vi "Remove Section.vi"(7 "Section Name":string, 8 "error in (no error)":errorcluster, 11 "Config in":refnum<class "LabVIEW-Config.lvclass">) -> (0 "error out":errorcluster, 2 "Section Found?":bool, 3 "Config out":refnum<class "LabVIEW-Config.lvclass">)   [LabVIEW 2017, in "LabVIEW-Config.lvlib" / "LabVIEW-Config.lvclass"]
uses:
  LabVIEW-Config.lvclass
  LabVIEW-Config.lvclass/LabVIEW-Config.ctl
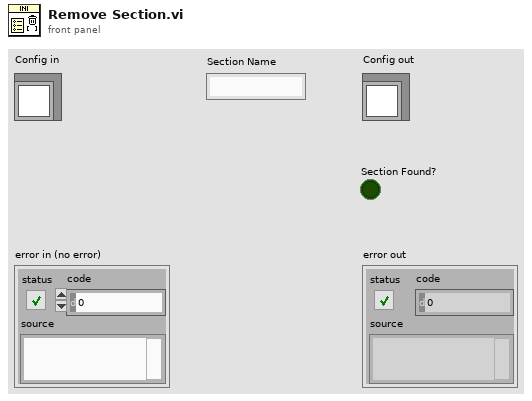
[diagram p1: front panel]
types:
  T1 = typedef "LabVIEW-Config.lvlib/LabVIEW-Config.lvclass/LineToken.ctl" = enum8{"comment", "section", "key", "more"}
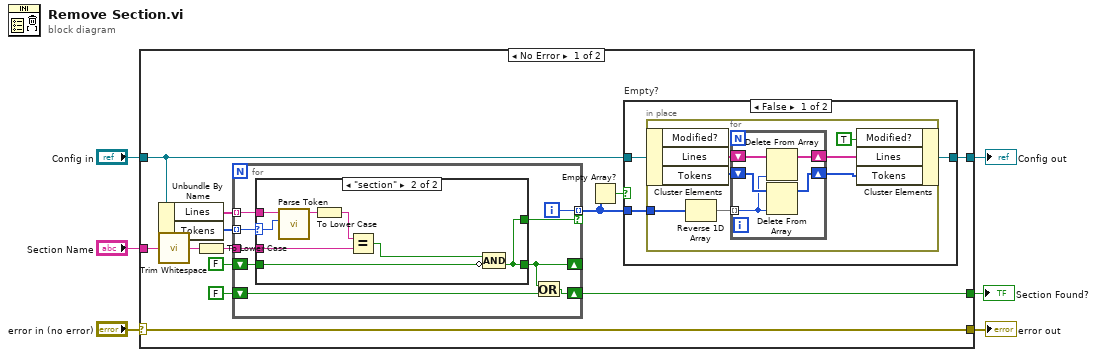
[diagram p0: block diagram]
diagram:
  n1 = case shown="No Error" "error in (no error)" {
    selector: "error in (no error)" -> [w17 w55]
    tunnel: "Config in" -> [w10 w54]
    tunnel: [w17 w55] -> w5
    tunnel: [w11 w54] -> w3
    tunnel: "Section Name" -> [w16 _]
    tunnel: [w12 _] -> w1
    frame No Error {
      n2 = Unbundle By Name(w10) -> ("Lines"=w18:string[], "Tokens"=w19:T1[])
      n3 = call <vilib>:"Trim Whitespace.vi"("string"=w16) -> ("trimmed string"=w7:string)  [unwired: 1 in]
      n4 = To Lower Case(string=w7) -> (all lower case string=w15:string)
      n5 = for {
        tunnel: w19 -> [w28] mode=indexing
        tunnel: w18 -> [w27] mode=indexing
        tunnel: [w20] -> w9 mode=indexing if=w24
        tunnel: w15 -> [w26]
        shift-right: [w23] -> _
        shift-left: FALSE -> [w25]
        shift-right: [w22] -> w12
        shift-left: FALSE -> [w21]
        i -> [w20]
        n6 = case shown="\"section\"" w28 {
          selector: w28 -> [_ w31]
          tunnel: w27 -> [_ w32]
          tunnel: w26 -> [_ w37]
          tunnel: [w29 w33] -> w23
          tunnel: w25 -> [w29 w35]
          tunnel: [w29 w33] -> w24
          frame Default {
          }
          frame "section" {
            n7 = call "Parse Token.vi"("Token"=w31, "Line"=w32) -> ("Name"=w30:string)  [unwired: 8 in, 1 out]
            n8 = To Lower Case(string=w30) -> (all lower case string=w36:string)
            n9 = Equal?(x=w36, y=w37) -> (x = y?=w34:bool)
            n10 = Compound Arithmetic op=AND(w34, invert w35) -> (w33:bool)
          }
        }
        n11 = Or(x=w23, y=w21) -> (x .or. y?=w22:bool)
      }
      n12 = Empty Array?(array=w9) -> (empty?=w8:bool)
      n13 = case "Empty?" shown="False" w8 {
        tunnel: [w40 w53] -> w11
        tunnel: w10 -> [w39 w53]
        tunnel: w9 -> [w38 _]
        frame False {
          n14 = in-place {
            in-place-border: w38 -> [w46]
            n15 = in-place-cluster #1(w39) -> ("Lines"=w45:string[], "Tokens"=w44:T1[])  [unwired: 1 out]
            n16 = Reverse 1D Array(array=w46) -> (reversed array=w41:i32[])
            n17 = for {
              shift-right: [w51] -> w42
              shift-left: w45 -> [w52]
              shift-right: [w48] -> w43
              shift-left: w44 -> [w50]
              tunnel: w41 -> [w49] mode=indexing
              n18 = Delete From Array(array=w52, index=w49) -> (array with subset deleted=w51:string[])  [unwired: 1 in, 1 out]
              n19 = Delete From Array(array=w50, index=w49) -> (array with subset deleted=w48:T1[])  [unwired: 1 in, 1 out]
            }
            n20 = in-place-cluster #1("Modified?"=TRUE, "Lines"=w42, "Tokens"=w43) -> (w40:refnum<class "LabVIEW-Config.lvclass">)
          }
        }
        frame True {
        }
      }
    }
    frame Error {
    }
  }
  "error out" <- w5
  "Config out" <- w3
  "Section Found?" <- w1
